vi "resistanceQuiry_RS458.vi"(0 "VISA resource name":refnum<visa-resource-name>="COM11", 11 "error in (no error)":errorcluster) -> (3 "resistMax":u32, 4 "dacMin":u32, 6 "dacMax":u32, 8 "Linear?":u32, 10 "Linear?":bool, 14 "RS485Type":u32, 15 "error out":errorcluster)   [LabVIEW 2018]
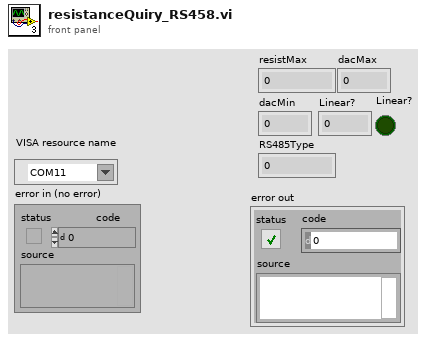
[diagram p1: front panel]
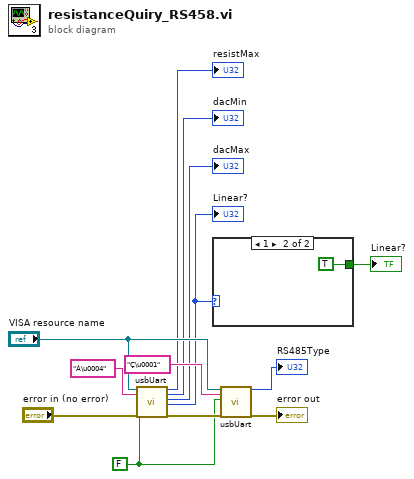
[diagram p0: block diagram]
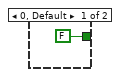
[diagram p2: hidden frame]
diagram:
  w1 = FALSE ("sdFeature")
  n1 = call "usbUart.vi"("VISA resource name"="VISA resource name", "write buffer"="Á\u0004", "sdFeature"=w1, "error in (no error)"="error in (no error)") -> ("number[0]"=→"resistMax":u32, "number[1]"=→"dacMin":u32, "number[2]"=→"dacMax":u32, "number[3]"=w5:u32, "error out"=w12:errorcluster)  [unwired: 11 out]
  "Linear?" <- w5
  n2 = case shown="1" w5 {
    tunnel: [FALSE TRUE] -> w4
    frame 0, Default {
    }
    frame 1 {
    }
  }
  "Linear?" <- w4
  n3 = call "usbUart.vi"("VISA resource name"="VISA resource name", "write buffer"="Ç\u0001", "sdFeature"=w1, "error in (no error)"=w12) -> ("number[0]"=→"RS485Type":u32, "error out"=→"error out":errorcluster)  [unwired: 14 out]
